vi "Truncate_cluster_general.vi"(1 "Length":i32=20, 2 "Cluster":cluster{"Array":dbl[], "Array 2":dbl[]}={"Array"=[2e-09, 5e-09, 1e-08, 2e-08, 5e-08, 1e-07, 2e-07, 5e-07, 1e-06, 2e-06, 5e-06, 1e-05, 2e-05, 5e-05, 0.0001, 0.0002, 0.0005, 0.001, 0.002, 0.005, 0.01, 0.02, 0.05, 0.1, 0.2, 0.5, 1.0], "Array 2"=[2e-09, 5e-09, 1e-08, 2e-08, 5e-08, 1e-07, 2e-07, 5e-07, 1e-06, 2e-06, 5e-06, 1e-05, 2e-05, 5e-05, 0.0001, 0.0002, 0.0005, 0.001, 0.002, 0.005, 0.01, 0.02, 0.05, 0.1, 0.2, 0.5, 1.0]}) -> (0 "Cluster 2":cluster{"Array":dbl[], "Array 2":dbl[]}={"Array"=[2e-09, 5e-09, 1e-08, 2e-08, 5e-08, 1e-07, 2e-07, 5e-07, 1e-06, 2e-06, 5e-06, 1e-05, 2e-05, 5e-05, 0.0001, 0.0002, 0.0005, 0.001, 0.002, 0.005, 0.01, 0.02, 0.05, 0.1, 0.2, 0.5, 1.0], "Array 2"=[2e-09, 5e-09, 1e-08, 2e-08, 5e-08, 1e-07, 2e-07, 5e-07, 1e-06, 2e-06, 5e-06, 1e-05, 2e-05, 5e-05, 0.0001, 0.0002, 0.0005, 0.001, 0.002, 0.005, 0.01, 0.02, 0.05, 0.1, 0.2, 0.5, 1.0]})   [LabVIEW 2015]
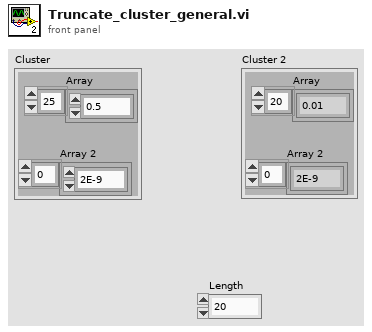
[diagram p1: front panel]
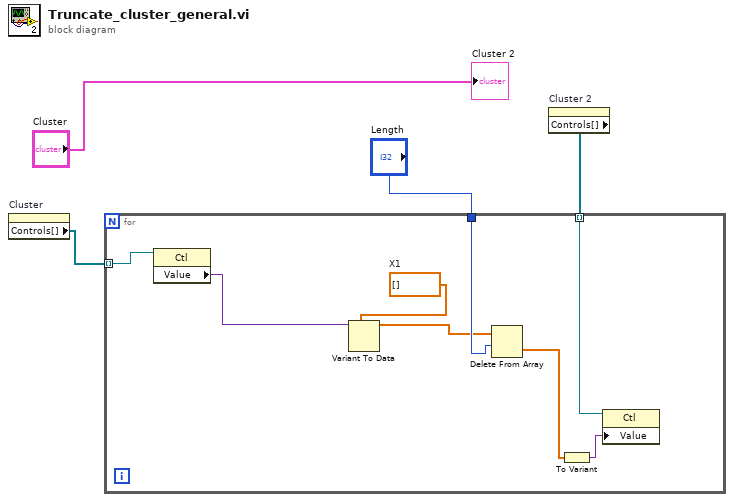
[diagram p0: block diagram]
diagram:
  n1 = property on="Cluster" class="Clust (strict)"() -> ("Controls[]"=w4:refnum<vi>[])  [unwired: 2 in, 2 out]
  n2 = property on="Cluster 2" class="Clust (strict)"() -> ("Controls[]"=w1:refnum<vi>[])  [unwired: 2 in, 2 out]
  n3 = for {
    tunnel: w4 -> [w11] mode=indexing
    tunnel: "Length" -> [w12]
    tunnel: w1 -> [w7] mode=indexing
    w9 = dbl[] []  # X1
    n4 = property class="Ctl"(reference=w11) -> ("Value"=w10:variant)  [unwired: 1 in, 2 out]
    n5 = Variant To Data(type=w9, Variant=w10) -> (data=w8:dbl[])  [unwired: 1 in, 1 out]
    n6 = Delete From Array(array=w8, length=w12) -> (deleted portion=w6:dbl[])  [unwired: 1 in, 1 out]
    n7 = To Variant(anything=w6) -> (Variant=w5:variant)
    n8 = property class="Ctl"(reference=w7, "Value"=w5) -> ()  [unwired: 1 in, 2 out]
  }
  "Cluster 2" <- "Cluster"
